vi "GPIB2400readvoltage.vi"() -> ()   [LabVIEW 2015]
panel:
  in  "address string":string="7"
  out "current":dbl format="%^.2e"
  in  "ms":u32 step=1
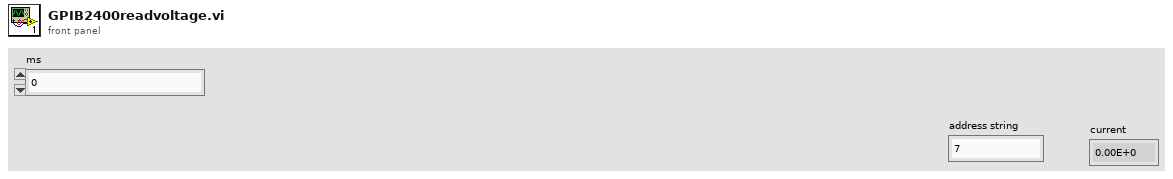
[diagram p1: front panel]
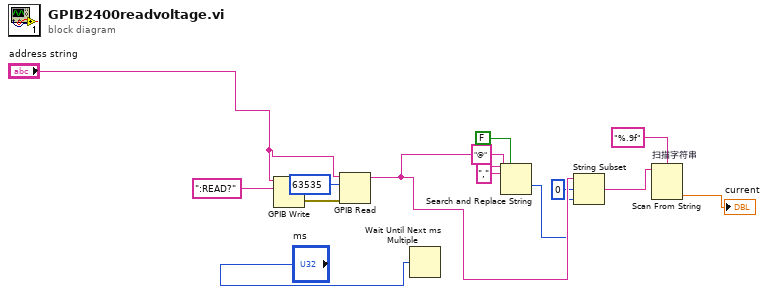
[diagram p0: block diagram]
diagram:
  n1 = GPIB Write(0:"address string", 1:":READ?" ("数据")) -> (6:w12:errorcluster)  [unwired: 3 in, 1 out]
  n2 = GPIB Read(0:"address string", 1:63535 ("字节总数"), 3:w12) -> (5:w7:string)  [unwired: 2 in, 2 out]
  n3 = Wait Until Next ms Multiple(millisecond multiple="ms") -> ()  [unwired: 1 out]
  n4 = Search and Replace String(replace all?=FALSE ("替换全部？(F)"), input string=w7, search string="," ("搜索字符串"), replace string="@" ("替换字符串(\"\")")) -> (offset past replacement=w5:i32)  [unwired: 4 in, 3 out]
  n5 = String Subset(string=w7, offset (0)=0 ("偏移量(0)"), length (rest)=w5) -> (substring=w4:string)
  n6 = Scan From String "扫描字符串"(format string="%.9f" ("格式字符串"), input string=w4) -> (output 1=→"current":dbl)  [unwired: 3 in, 3 out]
